vi "Init.vi"(8 "error in":errorcluster, 11 "Controller in":refnum<class "Controller.lvclass">) -> (0 "error out":errorcluster, 3 "Controller out":refnum<class "Controller.lvclass">)   [LabVIEW 2018, in "Controller.lvlib" / "Controller.lvclass"]
doc: "Launches the file writing Actors. This must bethe last to guarantee that the header is written properly."
uses:
  Controller.lvclass
  File Actor/File Actor.lvclass
  C:/Users/Labview/Documents/exscalabar_server/SuperActor/SuperActor.lvclass
  C:/Program Files (x86)/National Instruments/LabVIEW 2018/vi.lib/ActorFramework/Actor/Actor.lvclass
  Messages/Saving File MSG/Save Main File MSG.lvclass
  C:/Users/Labview/Documents/exscalabar_server/File Actor/Messages/Abstract/Saving File Message/Saving File Message.lvclass
  Messages/Execute Write Main/Exe Write Main.lvclass
  C:/Users/Labview/Documents/exscalabar_server/File Actor/Messages/Abstract/Exe Write/Exe Write.lvclass
  Controller.lvclass/Controller.ctl
  Messages/Execute Write Main/Exe Write Main.lvclass/Exe Write Main.ctl
  File Actor/File Actor.lvclass/File Actor.ctl
  SuperActor/SuperActor.lvclass/SuperActor.ctl
  Messages/Execute Write Main/Write MAP DVR.vi
  File Actor/Write Saving FIle MSG.vi
  File Actor/Write Exe Write.vi
  File Actor/Write Cfg Header.vi
  SuperActor/Write ID.vi
  SuperActor/Read Log Session.vi
  File Actor/Write Wait on Registration_.vi
  File Actor/Write Registration Complete.vi
  <userlib>/_Session Fwk/Session - Root.lvclass
  reusable/Session APIs/Session Log/System Log.lvclass
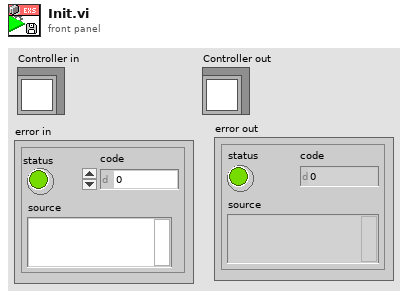
[diagram p1: front panel]
types:
  T1 = typedef "Session - Root.lvclass/Session Handle.ctl" = refnum<data-value>
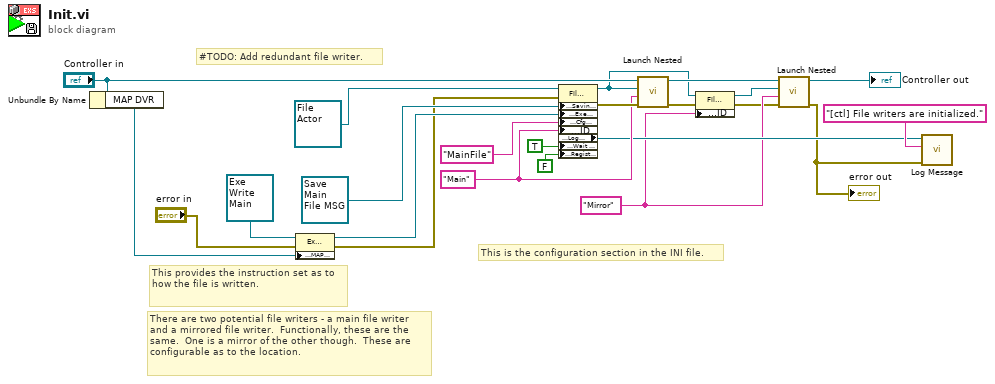
[diagram p0: block diagram]
diagram:
  w10 = "Mirror" ("ID")
  w19 = "Main" ("Cfg Header")
  # "This is the configuration section in the INI file."
  # "This provides the instruction set as to how the file is written."
  # "There are two potential file writers - a main file writer and a mirrored file writer.  Functionally, these are the same.  One is a mirror of the other though.  These are configurable as to the location."
  # "#TODO: Add redundant file writer."
  n1 = Unbundle By Name("Controller in") -> ("MAP DVR"=w15:refnum<data-value>)
  n2 = property class="Exe Write Main"(reference=refnum<class "Exe Write Main.lvclass"> refnum ("Controller.lvlib:Exe Write Main"), error in="error in", "Accessors:MAP DVR"=w15) -> (reference out=w17:refnum<class "Exe Write Main.lvclass">, error out=w3:errorcluster)
  n3 = property class="File Actor"(reference=refnum<class "File Actor.lvclass"> refnum ("File Library.lvlib:File Actor"), error in=w3, "Accessors:Saving FIle MSG"=refnum<class "Save Main File MSG.lvclass"> refnum ("Controller.lvlib:Save Main File MSG"), "Accessors:Exe Write"=w17, "Accessors:Cfg Header"="MainFile" ("Cfg Header"), "Accessors:ID"=w19, "Accessors:Wait on Registration_"=TRUE ("Wait on Registration_"), "Accessors:Registration Complete"=FALSE ("Registration Complete")) -> (reference out=w12:refnum<class "File Actor.lvclass">, error out=w20:errorcluster, "Accessors:Log Session"=w14:T1)
  n4 = call "Launch Nested.vi"("Error In"=w20, "ID"=w19, "Nested Actor"=w12, "Controller in"="Controller in") -> ("Error Out"=w7:errorcluster, "Controller out"=w13:refnum<class "Controller.lvclass">)  [unwired: 4 in, 2 out]
  n5 = property class="File Actor"(reference=w12, error in=w7, "Accessors:ID"=w10) -> (reference out=w11:refnum<class "File Actor.lvclass">, error out=w6:errorcluster)
  n6 = call "Launch Nested.vi"("Error In"=w6, "ID"=w10, "Nested Actor"=w11, "Controller in"=w13) -> ("Error Out"=w5:errorcluster, "Controller out"=→"Controller out":refnum<class "Controller.lvclass">)  [unwired: 4 in, 2 out]
  "error out" <- w5
  n7 = call "Log Message.vi"("error in"=w5, "MSG In"="[ctl] File writers are initialized.", "session in"=w14) -> ()  [unwired: 7 in, 2 out]
